vi "PCI-7390보드, 모션제어.vi"() -> ()   [LabVIEW 2014]
uses:
  <vilib>/Motion/FlexMotion/CustomControls/CustomControls.llb/AxisOrVectorSpace To Configure.flx
  <vilib>/Motion/FlexMotion/FunctionsVIs/StartStopMotion.llb/Start Motion (8 axes).flx
  <vilib>/Motion/FlexMotion/FunctionsVIs/StartStopMotion.llb/Stop Motion (8 axes).flx
panel:
  out "Filtered Velocity 2":dbl=600.0 format="%.2f"
  out "Per Axis H/W Status":T1
  out "Filtered Velocity":i32
  in  "정지":bool
  in  "Velocity (10000)":i32=36000
  # "Bit"
  # "Bit"
  # "0"
  # "8"
  # "9"
  # "1"
  # "10"
  # "2"
  # "11"
  # "3"
  # "4"
  # "12"
  # "13"
  # "5"
  # "14"
  # "6"
  # "15"
  # "7"
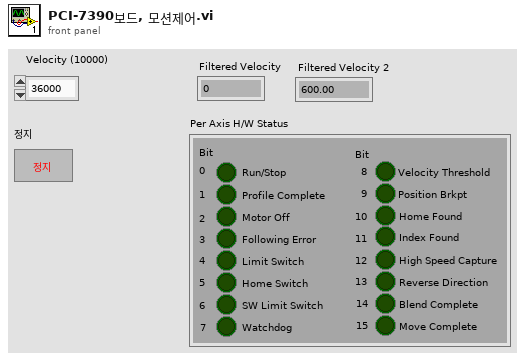
[diagram p1: front panel]
types:
  T1 = cluster{"Run/Stop":bool, "Profile Complete":bool, "Motor Off ":bool, "Following Error":bool, "Limit Switch":bool, "Home Switch":bool, "SW Limit Switch":bool, "Watchdog":bool, "Velocity Threshold":bool, "Position Brkpt":bool, "Home Found":bool, "Index Found":bool, "High Speed Capture":bool, "Reverse Direction":bool, "Blend Complete":bool, "Move Complete":bool}
  T2 = enum16{"Absolute Position", "Relative Position", "Velocity", "Relative to Cap Pos", "Modulus Position", "Absolute Contouring", "Relative Contouring"}
  T3 = typedef "AxisOrVectorSpace To Configure.flx" = u16
  T4 = typedef "Resource Out (Enum).flx" = u16
  T5 = typedef "Bd Id Out" = u8
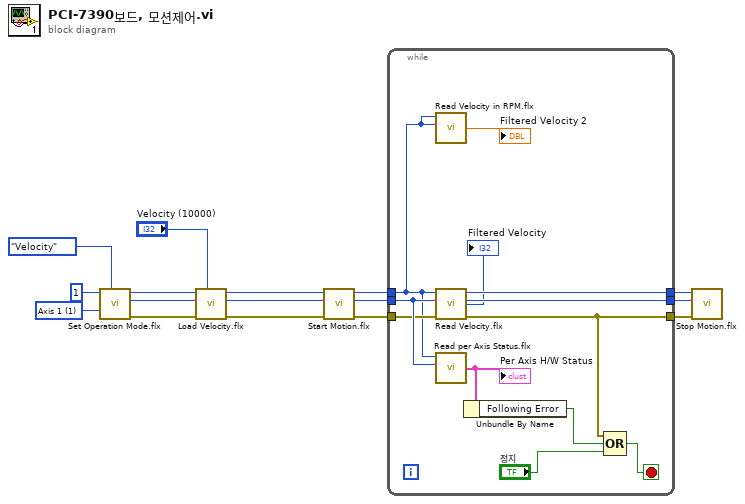
[diagram p0: block diagram]
diagram:
  w15 = T3 1 items=["Axis 1"=1, "Axis 2"=2, "Axis 3"=3, "Axis 4"=4, "Axis 5"=5, "Axis 6"=6, "Axis 7"=7, "Axis 8"=8, "Vector Space 1"=17, "Vector Space 2"=18, "Vector Space 3"=19, "Vector Space 4"=20] ("Axis or Vector Space")
  n1 = call <vilib>:"Set Operation Mode.flx"("Position Mode (Absolute)"=T2."Velocity", "Axis or Vector Space"=w15, "Board ID"=u8 1) -> ("error out"=w12:errorcluster, "Resource Output"=w13:T4, "Bd ID Out"=w14:T5)  [unwired: 3 in]
  n2 = call <vilib>:"Load Velocity.flx"("Velocity (10000)"="Velocity (10000)", "error in (no error)"=w12, "Axis or Vector Space"=w13, "Board ID"=w14) -> ("error out"=w8:errorcluster, "Resource Output"=w10:T4, "Bd ID Out"=w11:T5)  [unwired: 3 in]
  n3 = call-poly <vilib>:"Start Motion.flx"("error in (no error)"=w8, "Axis or Vector Space"=w10, "Board ID"=w11) -> ("error out"=w4:errorcluster, "Resource Output"=w5:T4, "Bd ID Out"=w6:T5)  [unwired: 3 in]
  n4 = while {
    tunnel: w6 -> [w18]
    tunnel: w5 -> [w26]
    tunnel: w4 -> [w19]
    tunnel: [w28] -> w3
    tunnel: [w27] -> w2
    tunnel: [w23] -> w1
    stop <- w20 stop-if-true
    n5 = call <vilib>:"Read Velocity in RPM.flx"("Axis or Vector Space"=w18, "Board ID"=w18) -> ("Filtered Velocity"=→"Filtered Velocity 2":dbl)  [unwired: 4 in, 3 out]
    n6 = call <vilib>:"Read Velocity.flx"("error in (no error)"=w19, "Axis or Vector Space"=w26, "Board ID"=w18) -> ("error out"=w23:errorcluster, "Resource Output"=w27:T4, "Bd ID Out"=w28:T5, "Filtered Velocity"=→"Filtered Velocity":i32)  [unwired: 3 in]
    n7 = call <vilib>:"Read per Axis Status.flx"("Axis"=w26, "Board ID"=w18) -> ("Per Axis H/W Status"=w24:T1)  [unwired: 4 in, 3 out]
    "Per Axis H/W Status" <- w24
    n8 = Unbundle By Name(w24) -> ("Following Error"=w22:bool)
    n9 = Compound Arithmetic op=OR(w23, w22, "정지") -> (w20:bool)
  }
  n10 = call-poly <vilib>:"Stop Motion.flx"("error in (no error)"=w1, "Axis or Vector Space"=w2, "Board ID"=w3) -> ()  [unwired: 4 in, 3 out]
